vi "Subscribe.vi"(6 "timeout (1000 ms)":i32=1000, 8 "error in (no error)":errorcluster, 9 "Packet ID (empty: Generate new)":u16 format="%04x", 10 "Topic Subscriptions":T3[](array[typedef]), 11 "MQTT_Base in":refnum<class "MQTT_Base.lvclass">) -> (0 "error out":errorcluster, 1 "SUBACK Packet ID":u16 format="%04x", 2 "Subscription Success":T1[](array[typedef]), 3 "MQTT_Base out":refnum<class "MQTT_Base.lvclass">)   [LabVIEW 2013, in "MQTT Base.lvlib" / "MQTT_Base.lvclass"]
uses:
  MQTT_Base.lvclass
  <vilib>/LabVIEW Open Source Project/MQTT Control Packets/Control Packets/SUBSCRIBE/Topic Subscription -- cluster.ctl
  <vilib>/LabVIEW Open Source Project/MQTT Control Packets/Control Packets/ControlPacket/QualityOfService -- enum.ctl
  <vilib>/LabVIEW Open Source Project/MQTT Control Packets/Control Packets/SUBACK/Subscription Success Code.ctl
  <vilib>/LabVIEW Open Source Project/MQTT Control Packets/Control Packets/ControlPacket/ControlPacket.lvclass/ControlPacket.ctl
  <vilib>/LabVIEW Open Source Project/MQTT Control Packets/Control Packets/SUBSCRIBE/SUBSCRIBE.lvclass
  <vilib>/LabVIEW Open Source Project/MQTT Control Packets/Control Packets/SUBACK/SUBACK.lvclass
  <vilib>/LabVIEW Open Source Project/MQTT Control Packets/Control Packets/ControlPacket/ControlPacket.lvclass
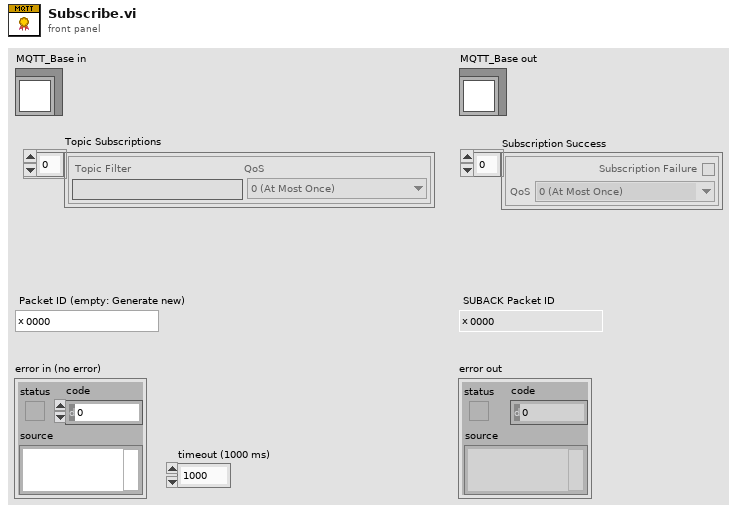
[diagram p1: front panel]
types:
  T1 = typedef "MQTT_Control_Packets.lvlib/SUBACK.lvclass/Subscription Success Code.ctl" = cluster{"Subscription Failure":bool, "QoS":T2}
  T2 = typedef "MQTT_Control_Packets.lvlib/ControlPacket.lvclass/QualityOfService -- enum.ctl" = enum16{"0 (At Most Once)", "1 (At Least Once)", "2 (Exactly Once)"}
  T3 = typedef "MQTT_Control_Packets.lvlib/SUBSCRIBE.lvclass/Topic Subscription -- cluster.ctl" = cluster{"Topic Filter":string, "QoS":T2}
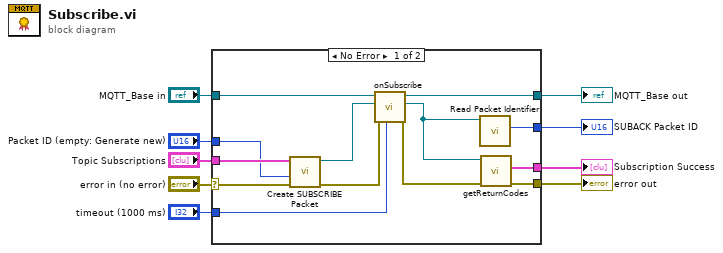
[diagram p0: block diagram]
diagram:
  n1 = case shown="No Error" "error in (no error)" {
    selector: "error in (no error)" -> [w18 w24]
    tunnel: [w14 w24] -> w8
    tunnel: [w21 w23] -> w6
    tunnel: "MQTT_Base in" -> [w22 w23]
    tunnel: "Topic Subscriptions" -> [w17 _]
    tunnel: [w16 _] -> w4
    tunnel: "timeout (1000 ms)" -> [w13 _]
    tunnel: "Packet ID (empty: Generate new)" -> [w12 _]
    tunnel: [w10 _] -> w1
    frame No Error {
      n2 = call <vilib>:"Create SUBSCRIBE Packet.vi"("error in (no error)"=w18, "Packet ID (empty: Generate new)"=w12, "Topic Subscriptions"=w17) -> ("error out"=w19:errorcluster, "SUBSCRIBE out"=w20:refnum<class "SUBSCRIBE.lvclass">)  [unwired: 6 in, 1 out]
      n3 = call-dynamic "onSubscribe.vi"("timeout (100ms)"=w13, "error in (no error)"=w19, "SUBSCRIBE"=w20, "MQTT_Base in"=w22) -> ("error out"=w15:errorcluster, "SUBACK"=w11:refnum<class "SUBACK.lvclass">, "MQTT_Base out"=w21:refnum<class "MQTT_Base.lvclass">)  [unwired: 4 in, 1 out]
      n4 = call <vilib>:"Read Packet Identifier.vi"("ControlPacket in"=w11) -> ("Packet Identifier"=w10:u16)  [unwired: 9 in, 1 out]
      n5 = call <vilib>:"getReturnCodes.vi"("error in (no error)"=w15, "SUBACK in"=w11) -> ("error out"=w14:errorcluster, "Subscription Success"=w16:T1[])  [unwired: 7 in, 1 out]
    }
    frame Error {
    }
  }
  "error out" <- w8
  "MQTT_Base out" <- w6
  "Subscription Success" <- w4
  "SUBACK Packet ID" <- w1
